vi "Read configuration.vi"(8 "error in":errorcluster, 11 "ActiveFrontEndModule editor node in":refnum<class "ActiveFrontEndModule editor node.lvclass">) -> (0 "error out":errorcluster, 2 "configuration":refnum<class "NISE_CEF_serializable configuration.lvclass">, 3 "ActiveFrontEndModule editor node out":refnum<class "ActiveFrontEndModule editor node.lvclass">)   [LabVIEW 2017, in "ActiveFrontEndModule editor node.lvclass"]
uses:
  ActiveFrontEndModule editor node.lvclass
  <vilib>/NI/Configuration Framework/serializable configuration/NISE_CEF_serializable configuration.lvclass
  ActiveFrontEndModule editor node.lvclass/ActiveFrontEndModule editor node.ctl
  module/configuration/ActiveFrontEndModule configuration.lvclass
  C:/Program Files (x86)/National Instruments/LabVIEW 2017/vi.lib/NI/Configuration Framework/serializable configuration/NISE_CEF_serializable configuration.lvclass
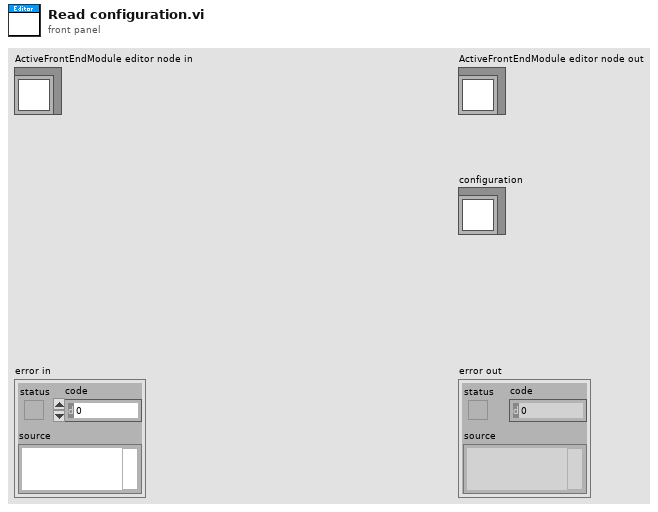
[diagram p1: front panel]
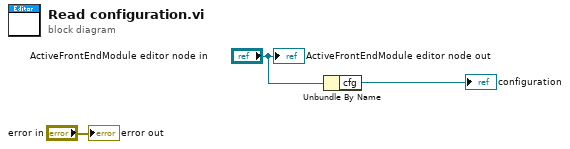
[diagram p0: block diagram]
diagram:
  n1 = Unbundle By Name("ActiveFrontEndModule editor node in") -> ("cfg"=→"configuration":refnum<class "ActiveFrontEndModule configuration.lvclass">)
  "error out" <- "error in"
  "ActiveFrontEndModule editor node out" <- "ActiveFrontEndModule editor node in"
